vi "Position.vi"(0 "Position":dbl[][](array[numeric])) -> (6 "Position (output)":dbl[][](array[numeric]), 7 "Normalized Position":dbl[][](array[numeric]), 8 "RMS":dbl[][](array[numeric]), 9 "Pos, Neg increments Position":dbl[][](array[numeric]))   [LabVIEW 2020]
uses:
  <vilib>/Analysis/baseanly.llb/Mean (DBL).vi
  <vilib>/Analysis/5stat.llb/RMS (DBL).vi
  <vilib>/Analysis/NI_AALBase.lvlib
  <vilib>/Analysis/NI_AALPro.lvlib
panel:
  out "Positive, neg increments position":dbl[](array[numeric])
  out "Wrist Retraction":dbl
  out "Negative increments 6":dbl[](array[numeric])
  out "Wrist Protraction":dbl
  out "Positive increments 6":dbl[](array[numeric])
  out "Wrist Drop":dbl
  out "Negative increments 5":dbl[](array[numeric])
  out "Wrist Lift":dbl
  out "Positive increments 5":dbl[](array[numeric])
  out "Elbow Retraction":dbl
  out "Negative increments 4":dbl[](array[numeric])
  out "Elbow Protraction":dbl
  out "Positive increments 4":dbl[](array[numeric])
  out "Elbow Drop":dbl
  out "Negative increments 3":dbl[](array[numeric])
  out "Elbow Lift":dbl
  out "Positive increments 3":dbl[](array[numeric])
  out "Shoulder Retraction":dbl
  out "Negative increments 2":dbl[](array[numeric])
  out "Shoulder Protraction":dbl
  out "Positive increments 2":dbl[](array[numeric])
  out "Shoulder Drop":dbl
  out "Negative increments":dbl[](array[numeric])
  out "Shoulder Lift":dbl
  out "Positive increments":dbl[](array[numeric])
  out "size(s)":i32[](array[numeric])
  out "output array":dbl[](array[numeric])
  out "Array":dbl[][](array[numeric])
  out "Step Y (horizontal)":dbl[](graph)
  out "Step X (vertical)":dbl[](graph)
  out "Wrist X (vertical) 2":dbl[](graph)
  out "Wrist Y (horizontal) 2":dbl[](graph)
  out "Elbow X (vertical)  2":dbl[](graph)
  out "Elbow Y (horizontal)  2":dbl[](graph)
  out "Lower shoulder  X (vertical)  2":dbl[](graph)
  out "Lower shoulder Y (horizontal)  2":dbl[](graph)
  out "Upper shoulder X (vertical) 2":dbl[](graph)
  out "Upper shoulder Y (horizontal) 2":dbl[](graph)
  out "Wrist X (vertical)":dbl[](graph)
  out "Wrist Y (horizontal)":dbl[](graph)
  out "Elbow X (vertical)":dbl[](graph)
  out "Elbow Y (horizontal)":dbl[](graph)
  out "Lower shoulder  X (vertical)":dbl[](graph)
  out "Lower shoulder Y (horizontal)":dbl[](graph)
  out "Upper shoulder X (vertical)":dbl[](graph)
  out "Upper shoulder Y (horizontal)":dbl[](graph)
  # "Displacement and time kinematics"
  # "Upper Shoulder - Vertical"
  # "Upper shoulder - Horizontal"
  # "Lower Shoulder - Vertical"
  # "Lower shoulder - Horizontal"
  # "Elbow - Vertical"
  # "Elbow - Horizontal"
  # "Wrist - Vertical"
  # "Wrist - Horizontal"
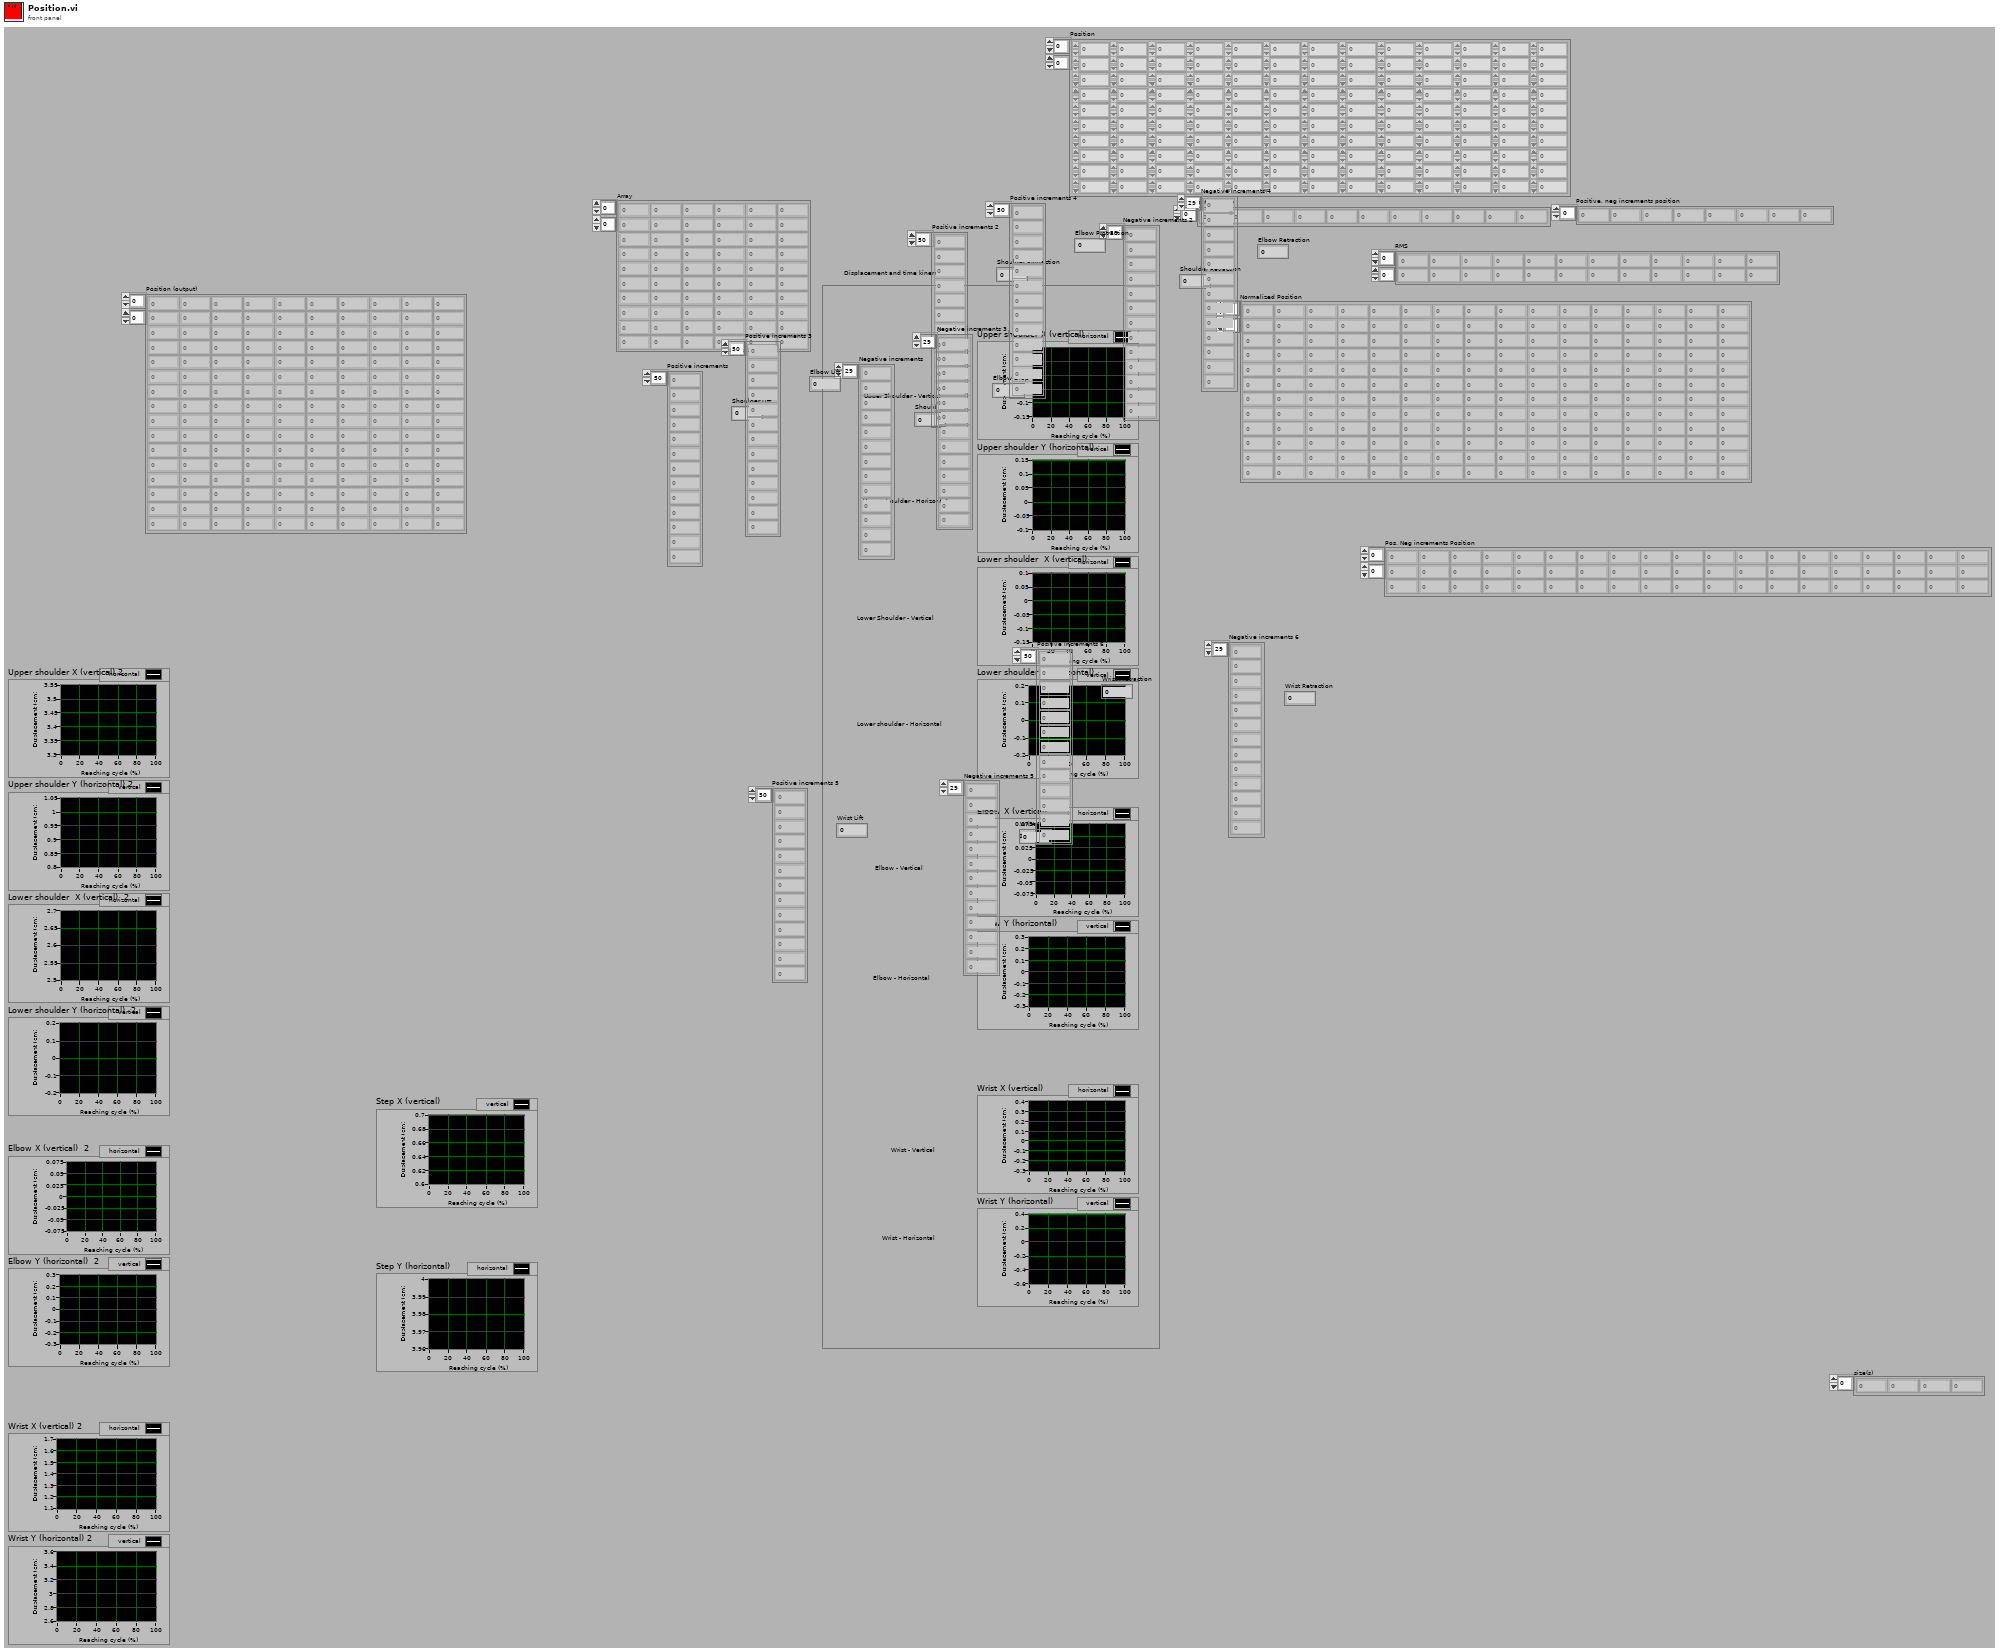
[diagram p1: front panel]
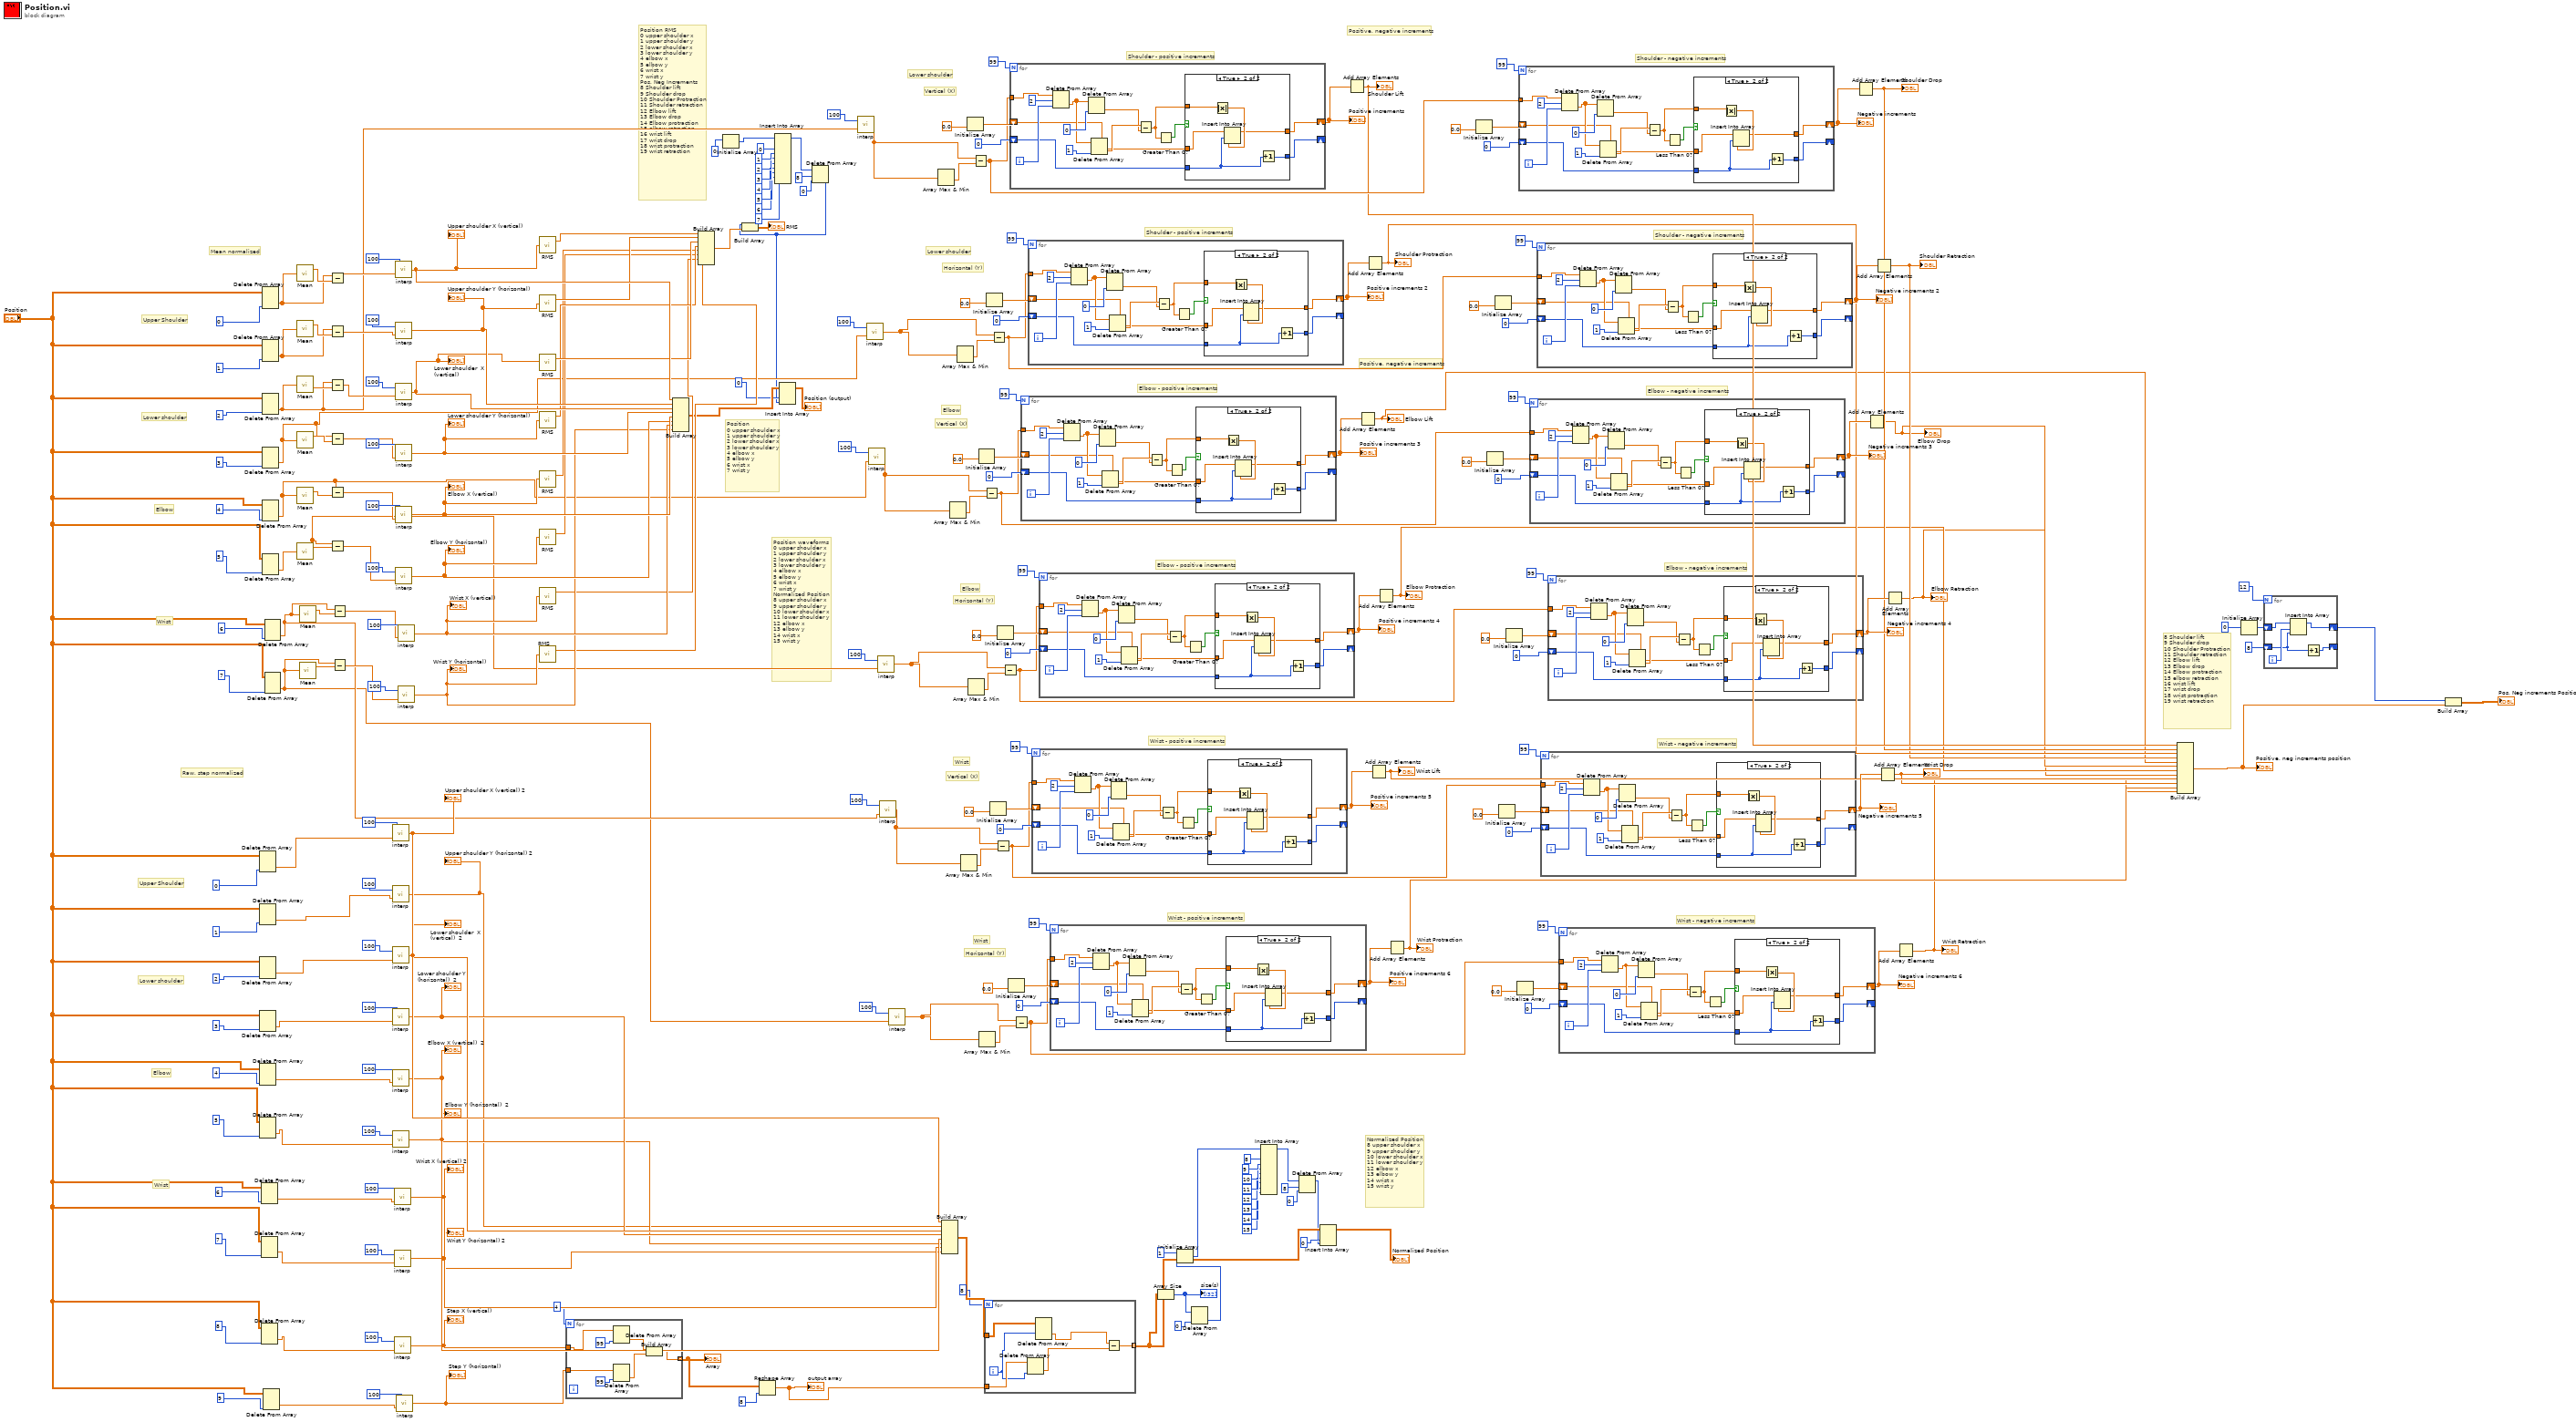
[diagram p0: block diagram]
diagram:
  # "Position waveforms\n0 upper shoulder x\n1 upper shoulder y\n2 lower shoulder x\n3 lower shoulder y\n4 elbow x\n5 elbow y\n6 wrist x\n7 wrist y\nNormalized Position\n8 upper shoulder x\n9 upper shoulder y\n10 lower shoulder x\n11 lower shoulder y\n12 elbow x\n13 elbow y\n14 wrist x\n15 wrist y"
  # "Position RMS\n0 upper shoulder x\n1 upper shoulder y\n2 lower shoulder x\n3 lower shoulder y\n4 elbow x\n5 elbow y\n6 wrist x\n7 wrist y\nPos, Neg Increments\n8 Shoulder lift\n9 Shoulder drop\n10 Shoulder Protraction\n11 Shoulder retraction\n12 Elbow lift\n13 Elbow drop\n14 Elbow protraction\n15 elbow retraction\n16 wrist lift\n17 wrist drop\n18 wrist protraction\n19 wrist retraction"
  # "8 Shoulder lift\n9 Shoulder drop\n10 Shoulder Protraction\n11 Shoulder retraction\n12 Elbow lift\n13 Elbow drop\n14 Elbow protraction\n15 elbow retraction\n16 wrist lift\n17 wrist drop\n18 wrist protraction\n19 wrist retraction"
  # "Wrist"
  # "Horizontal (Y)"
  # "Wrist - negative increments"
  # "Wrist - positive increments"
  # "Vertical (X)"
  # "Wrist - negative increments"
  # "Wrist - positive increments"
  # "Elbow"
  # "Horizontal (Y)"
  # "Elbow - negative increments"
  # "Elbow - positive increments"
  # "Vertical (X)"
  # "Elbow - negative increments"
  # "Elbow - positive increments"
  # "Positive, negative increments"
  # "Horizontal (Y)"
  # "Shoulder - negative increments"
  # "Shoulder - positive increments"
  # "Lower shoulder"
  # "Vertical (X)"
  # "Shoulder - negative increments"
  # "Shoulder - positive increments"
  # "Wrist"
  # "Elbow"
  # "Lower shoulder"
  # "Positive, negative increments"
  # "Normalized Position\n8 upper shoulder x\n9 upper shoulder y\n10 lower shoulder x\n11 lower shoulder y\n12 elbow x\n13 elbow y\n14 wrist x\n15 wrist y"
  # "Wrist"
  # "Elbow"
  # "Lower shoulder"
  # "Upper Shoulder"
  # "Raw, step normalized"
  # "Mean normalized"
  # "Wrist"
  # "Position\n0 upper shoulder x\n1 upper shoulder y\n2 lower shoulder x\n3 lower shoulder y\n4 elbow x\n5 elbow y\n6 wrist x\n7 wrist y"
  # "Elbow"
  # "Lower shoulder"
  # "Upper Shoulder"
  n1 = Delete From Array(array="Position", index (col)=0) -> (deleted portion=w189:dbl[])  [unwired: 2 in, 1 out]
  n2 = Delete From Array(array="Position", index (col)=1) -> (deleted portion=w188:dbl[])  [unwired: 2 in, 1 out]
  n3 = Delete From Array(array="Position", index (col)=2) -> (deleted portion=w187:dbl[])  [unwired: 2 in, 1 out]
  n4 = Delete From Array(array="Position", index (col)=3) -> (deleted portion=w186:dbl[])  [unwired: 2 in, 1 out]
  n5 = Delete From Array(array="Position", index (col)=4) -> (deleted portion=w185:dbl[])  [unwired: 2 in, 1 out]
  n6 = Delete From Array(array="Position", index (col)=5) -> (deleted portion=w184:dbl[])  [unwired: 2 in, 1 out]
  n7 = Delete From Array(array="Position", index (col)=6) -> (deleted portion=w183:dbl[])  [unwired: 2 in, 1 out]
  n8 = Delete From Array(array="Position", index (col)=7) -> (deleted portion=w182:dbl[])  [unwired: 2 in, 1 out]
  n9 = Delete From Array(array="Position", index (col)=8) -> (deleted portion=w176:dbl[])  [unwired: 2 in, 1 out]
  n10 = Delete From Array(array="Position", index (col)=0) -> (deleted portion=w131:dbl[])  [unwired: 2 in, 1 out]
  n11 = Delete From Array(array="Position", index (col)=1) -> (deleted portion=w222:dbl[])  [unwired: 2 in, 1 out]
  n12 = Delete From Array(array="Position", index (col)=2) -> (deleted portion=w114:dbl[])  [unwired: 2 in, 1 out]
  n13 = Delete From Array(array="Position", index (col)=3) -> (deleted portion=w99:dbl[])  [unwired: 2 in, 1 out]
  n14 = Delete From Array(array="Position", index (col)=4) -> (deleted portion=w69:dbl[])  [unwired: 2 in, 1 out]
  n15 = Delete From Array(array="Position", index (col)=5) -> (deleted portion=w68:dbl[])  [unwired: 2 in, 1 out]
  n16 = Delete From Array(array="Position", index (col)=9) -> (deleted portion=w175:dbl[])  [unwired: 2 in, 1 out]
  n17 = Delete From Array(array="Position", index (col)=6) -> (deleted portion=w39:dbl[])  [unwired: 2 in, 1 out]
  n18 = Delete From Array(array="Position", index (col)=7) -> (deleted portion=w38:dbl[])  [unwired: 2 in, 1 out]
  n19 = call-poly <vilib>:"Mean.vi"("X"=w131) -> ("mean"=w242:dbl)  [unwired: 1 out]
  n20 = call-poly <vilib>:"Mean.vi"("X"=w222) -> ("mean"=w243:dbl)  [unwired: 1 out]
  n21 = call-poly <vilib>:"Mean.vi"("X"=w114) -> ("mean"=w238:dbl)  [unwired: 1 out]
  n22 = call-poly <vilib>:"Mean.vi"("X"=w99) -> ("mean"=w239:dbl)  [unwired: 1 out]
  n23 = call-poly <vilib>:"Mean.vi"("X"=w69) -> ("mean"=w234:dbl)  [unwired: 1 out]
  n24 = call-poly <vilib>:"Mean.vi"("X"=w68) -> ("mean"=w235:dbl)  [unwired: 1 out]
  n25 = call-poly <vilib>:"Mean.vi"("X"=w39) -> ("mean"=w218:dbl)  [unwired: 1 out]
  n26 = call-poly <vilib>:"Mean.vi"("X"=w38) -> ("mean"=w219:dbl)  [unwired: 1 out]
  n27 = Subtract(x=w131, y=w242) -> (x-y=w130:dbl[])
  n28 = Subtract(x=w222, y=w243) -> (x-y=w227:dbl[])
  n29 = Subtract(x=w114, y=w238) -> (x-y=w226:dbl[])
  n30 = Subtract(x=w99, y=w239) -> (x-y=w225:dbl[])
  n31 = Subtract(x=w69, y=w234) -> (x-y=w224:dbl[])
  n32 = Subtract(x=w68, y=w235) -> (x-y=w223:dbl[])
  n33 = Subtract(x=w39, y=w218) -> (x-y=w215:dbl[])
  n34 = Subtract(x=w38, y=w219) -> (x-y=w214:dbl[])
  n35 = call "interp.vi"("first subarray"=w189, "nFRAMES"=100) -> ("emgInterp"=w201:dbl[])
  "Upper shoulder X (vertical) 2" <- w201
  n36 = call "interp.vi"("first subarray"=w188, "nFRAMES"=100) -> ("emgInterp"=w196:dbl[])
  "Upper shoulder Y (horizontal) 2" <- w196
  n37 = call "interp.vi"("first subarray"=w187, "nFRAMES"=100) -> ("emgInterp"=w200:dbl[])
  "Lower shoulder  X (vertical)  2" <- w200
  n38 = call "interp.vi"("first subarray"=w186, "nFRAMES"=100) -> ("emgInterp"=w199:dbl[])
  "Lower shoulder Y (horizontal)  2" <- w199
  n39 = call "interp.vi"("first subarray"=w185, "nFRAMES"=100) -> ("emgInterp"=w198:dbl[])
  "Elbow X (vertical)  2" <- w198
  n40 = call "interp.vi"("first subarray"=w184, "nFRAMES"=100) -> ("emgInterp"=w197:dbl[])
  "Elbow Y (horizontal)  2" <- w197
  n41 = call "interp.vi"("first subarray"=w183, "nFRAMES"=100) -> ("emgInterp"=w191:dbl[])
  "Wrist X (vertical) 2" <- w191
  n42 = call "interp.vi"("first subarray"=w182, "nFRAMES"=100) -> ("emgInterp"=w190:dbl[])
  "Wrist Y (horizontal) 2" <- w190
  n43 = call "interp.vi"("first subarray"=w176, "nFRAMES"=100) -> ("emgInterp"=w173:dbl[])
  "Step X (vertical)" <- w173
  n44 = call "interp.vi"("first subarray"=w130, "nFRAMES"=100) -> ("emgInterp"=w147:dbl[])
  "Upper shoulder X (vertical)" <- w147
  n45 = call "interp.vi"("first subarray"=w227, "nFRAMES"=100) -> ("emgInterp"=w146:dbl[])
  "Upper shoulder Y (horizontal)" <- w146
  n46 = call "interp.vi"("first subarray"=w226, "nFRAMES"=100) -> ("emgInterp"=w145:dbl[])
  "Lower shoulder  X (vertical)" <- w145
  n47 = call "interp.vi"("first subarray"=w225, "nFRAMES"=100) -> ("emgInterp"=w144:dbl[])
  "Lower shoulder Y (horizontal)" <- w144
  n48 = call "interp.vi"("first subarray"=w224, "nFRAMES"=100) -> ("emgInterp"=w143:dbl[])
  "Elbow X (vertical)" <- w143
  n49 = call "interp.vi"("first subarray"=w223, "nFRAMES"=100) -> ("emgInterp"=w142:dbl[])
  "Elbow Y (horizontal)" <- w142
  n50 = call "interp.vi"("first subarray"=w175, "nFRAMES"=100) -> ("emgInterp"=w172:dbl[])
  "Step Y (horizontal)" <- w172
  n51 = call "interp.vi"("first subarray"=w215, "nFRAMES"=100) -> ("emgInterp"=w141:dbl[])
  "Wrist X (vertical)" <- w141
  n52 = call "interp.vi"("first subarray"=w214, "nFRAMES"=100) -> ("emgInterp"=w140:dbl[])
  "Wrist Y (horizontal)" <- w140
  n53 = call-poly <vilib>:"RMS.vi"("X"=w147) -> ("rms value"=w139:dbl)  [unwired: 1 out]
  n54 = call-poly <vilib>:"RMS.vi"("X"=w146) -> ("rms value"=w138:dbl)  [unwired: 1 out]
  n55 = call-poly <vilib>:"RMS.vi"("X"=w145) -> ("rms value"=w137:dbl)  [unwired: 1 out]
  n56 = call-poly <vilib>:"RMS.vi"("X"=w144) -> ("rms value"=w136:dbl)  [unwired: 1 out]
  n57 = call-poly <vilib>:"RMS.vi"("X"=w143) -> ("rms value"=w135:dbl)  [unwired: 1 out]
  n58 = call-poly <vilib>:"RMS.vi"("X"=w142) -> ("rms value"=w134:dbl)  [unwired: 1 out]
  n59 = call-poly <vilib>:"RMS.vi"("X"=w141) -> ("rms value"=w133:dbl)  [unwired: 1 out]
  n60 = call-poly <vilib>:"RMS.vi"("X"=w140) -> ("rms value"=w132:dbl)  [unwired: 1 out]
  n61 = for {
    N: 4 -> [_]
    tunnel: w173 -> [w247]
    tunnel: [w248] -> w170 mode=indexing
    tunnel: w172 -> [w246]
    n62 = Delete From Array(array=w247, index=99) -> (deleted portion=w250:dbl)  [unwired: 1 in, 1 out]
    n63 = Delete From Array(array=w246, index=99) -> (deleted portion=w249:dbl)  [unwired: 1 in, 1 out]
    n64 = Build Array(w250, w249) -> (w248:dbl[])
  }
  "Array" <- w170
  n65 = Build Array(w147, w146, w145, w144, w143, w142, w141, w140) -> (w18:dbl[][])
  n66 = Build Array(w139, w138, w137, w136, w135, w134, w133, w132) -> (w129:dbl[])
  n67 = Initialize Array(0) -> (w3:i32[])  [unwired: 1 in]
  n68 = Reshape Array(w170, 8) -> (w168:dbl[])
  "output array" <- w168
  n69 = Insert Into Array(array=w3, new element #1=0, new element #2=1, new element #3=2, new element #4=3, new element #5=4, new element #6=5, new element #7=6, new element #8=7) -> (w7:i32[])  [unwired: 1 in]
  n70 = Delete From Array(array=w7, length=8, index=0) -> (deleted portion=w1:i32[])  [unwired: 1 out]
  n71 = Build Array(w1, w129) -> (→"RMS":dbl[][])
  n72 = Insert Into Array(array=w18, index (col)=0, new element=w1) -> (→"Position (output)":dbl[][])  [unwired: 1 in]
  n73 = call "interp.vi"("first subarray"=w114, "nFRAMES"=100) -> ("emgInterp"=w113:dbl[])
  n74 = call "interp.vi"("first subarray"=w99, "nFRAMES"=100) -> ("emgInterp"=w98:dbl[])
  n75 = call "interp.vi"("first subarray"=w69, "nFRAMES"=100) -> ("emgInterp"=w84:dbl[])
  n76 = call "interp.vi"("first subarray"=w68, "nFRAMES"=100) -> ("emgInterp"=w70:dbl[])
  n77 = call "interp.vi"("first subarray"=w39, "nFRAMES"=100) -> ("emgInterp"=w54:dbl[])
  n78 = call "interp.vi"("first subarray"=w38, "nFRAMES"=100) -> ("emgInterp"=w40:dbl[])
  n79 = Array Max & Min(array=w113) -> (min value=w127:dbl)  [unwired: 3 out]
  n80 = Build Array(w201, w196, w200, w199, w198, w197, w191, w190) -> (w169:dbl[][])
  n81 = Array Max & Min(array=w84) -> (min value=w97:dbl)  [unwired: 3 out]
  n82 = Array Max & Min(array=w98) -> (min value=w112:dbl)  [unwired: 3 out]
  n83 = Array Max & Min(array=w54) -> (min value=w67:dbl)  [unwired: 3 out]
  n84 = Initialize Array(0.0) -> (w125:dbl[])  [unwired: 1 in]
  n85 = Array Max & Min(array=w70) -> (min value=w83:dbl)  [unwired: 3 out]
  n86 = Subtract(x=w113, y=w127) -> (x-y=w116:dbl[])
  n87 = Initialize Array(0.0) -> (w95:dbl[])  [unwired: 1 in]
  n88 = Array Max & Min(array=w40) -> (min value=w53:dbl)  [unwired: 3 out]
  n89 = Subtract(x=w84, y=w97) -> (x-y=w86:dbl[])
  n90 = for {
    N: 8 -> [_]
    tunnel: w169 -> [w258]
    tunnel: [w256] -> w149 mode=indexing
    tunnel: w168 -> [w255]
    i -> [w254]
    n91 = Delete From Array(array=w255, index=w254) -> (deleted portion=w253:dbl)  [unwired: 1 in, 1 out]
    n92 = Delete From Array(array=w258, index (row)=w254) -> (deleted portion=w257:dbl[])  [unwired: 2 in, 1 out]
    n93 = Subtract(x=w257, y=w253) -> (x-y=w256:dbl[])
  }
  n94 = Initialize Array(0.0) -> (w110:dbl[])  [unwired: 1 in]
  n95 = Initialize Array(0.0) -> (w65:dbl[])  [unwired: 1 in]
  n96 = Subtract(x=w98, y=w112) -> (x-y=w101:dbl[])
  n97 = Subtract(x=w54, y=w67) -> (x-y=w56:dbl[])
  n98 = Initialize Array(0.0) -> (w81:dbl[])  [unwired: 1 in]
  n99 = Subtract(x=w70, y=w83) -> (x-y=w72:dbl[])
  n100 = Initialize Array(0.0) -> (w51:dbl[])  [unwired: 1 in]
  n101 = for {
    N: 99 -> [_]
    shift-right: [w259] -> _
    shift-left: 0 -> [w261]
    shift-right: [w260] -> w122
    shift-left: w125 -> [w262]
    tunnel: w116 -> [w272]
    i -> [w271]
    n102 = Delete From Array(array=w272, length=2, index=w271) -> (deleted portion=w267:dbl[])  [unwired: 1 out]
    n103 = Delete From Array(array=w267, index=0) -> (deleted portion=w265:dbl)  [unwired: 1 in, 1 out]
    n104 = Delete From Array(array=w267, index=1) -> (deleted portion=w266:dbl)  [unwired: 1 in, 1 out]
    n105 = Subtract(x=w266, y=w265) -> (x-y=w263:dbl)
    n106 = Greater Than 0?(x=w263) -> (x > 0?=w264:bool)
    n107 = case shown="True" w264 {
      tunnel: w263 -> [_ w280]
      tunnel: w262 -> [w274 w279]
      tunnel: w261 -> [w273 w276]
      tunnel: [w274 w277] -> w260
      tunnel: [w273 w275] -> w259
      frame False {
      }
      frame True {
        n108 = Absolute Value(x=w280) -> (abs(x)=w278:dbl)
        n109 = Insert Into Array(array=w279, index=w276, new element=w278) -> (w277:dbl[])
        n110 = Increment(x=w276) -> (x+1=w275:i32)
      }
    }
  }
  "Positive increments" <- w122
  n111 = Subtract(x=w40, y=w53) -> (x-y=w42:dbl[])
  n112 = for {
    N: 99 -> [_]
    shift-right: [w281] -> _
    shift-left: 0 -> [w283]
    shift-right: [w282] -> w92
    shift-left: w95 -> [w284]
    tunnel: w86 -> [w294]
    i -> [w293]
    n113 = Delete From Array(array=w294, length=2, index=w293) -> (deleted portion=w289:dbl[])  [unwired: 1 out]
    n114 = Delete From Array(array=w289, index=0) -> (deleted portion=w287:dbl)  [unwired: 1 in, 1 out]
    n115 = Delete From Array(array=w289, index=1) -> (deleted portion=w288:dbl)  [unwired: 1 in, 1 out]
    n116 = Subtract(x=w288, y=w287) -> (x-y=w285:dbl)
    n117 = Greater Than 0?(x=w285) -> (x > 0?=w286:bool)
    n118 = case shown="True" w286 {
      tunnel: w285 -> [_ w302]
      tunnel: w284 -> [w296 w301]
      tunnel: w283 -> [w295 w298]
      tunnel: [w296 w299] -> w282
      tunnel: [w295 w297] -> w281
      frame False {
      }
      frame True {
        n119 = Absolute Value(x=w302) -> (abs(x)=w300:dbl)
        n120 = Insert Into Array(array=w301, index=w298, new element=w300) -> (w299:dbl[])
        n121 = Increment(x=w298) -> (x+1=w297:i32)
      }
    }
  }
  "Positive increments 3" <- w92
  n122 = for {
    N: 99 -> [_]
    shift-right: [w303] -> _
    shift-left: 0 -> [w305]
    shift-right: [w304] -> w107
    shift-left: w110 -> [w306]
    tunnel: w101 -> [w316]
    i -> [w315]
    n123 = Delete From Array(array=w316, length=2, index=w315) -> (deleted portion=w311:dbl[])  [unwired: 1 out]
    n124 = Delete From Array(array=w311, index=0) -> (deleted portion=w309:dbl)  [unwired: 1 in, 1 out]
    n125 = Delete From Array(array=w311, index=1) -> (deleted portion=w310:dbl)  [unwired: 1 in, 1 out]
    n126 = Subtract(x=w310, y=w309) -> (x-y=w307:dbl)
    n127 = Greater Than 0?(x=w307) -> (x > 0?=w308:bool)
    n128 = case shown="True" w308 {
      tunnel: w307 -> [_ w324]
      tunnel: w306 -> [w318 w323]
      tunnel: w305 -> [w317 w320]
      tunnel: [w318 w321] -> w304
      tunnel: [w317 w319] -> w303
      frame False {
      }
      frame True {
        n129 = Absolute Value(x=w324) -> (abs(x)=w322:dbl)
        n130 = Insert Into Array(array=w323, index=w320, new element=w322) -> (w321:dbl[])
        n131 = Increment(x=w320) -> (x+1=w319:i32)
      }
    }
  }
  "Positive increments 2" <- w107
  n132 = for {
    N: 99 -> [_]
    shift-right: [w325] -> _
    shift-left: 0 -> [w327]
    shift-right: [w326] -> w62
    shift-left: w65 -> [w328]
    tunnel: w56 -> [w338]
    i -> [w337]
    n133 = Delete From Array(array=w338, length=2, index=w337) -> (deleted portion=w333:dbl[])  [unwired: 1 out]
    n134 = Delete From Array(array=w333, index=0) -> (deleted portion=w331:dbl)  [unwired: 1 in, 1 out]
    n135 = Delete From Array(array=w333, index=1) -> (deleted portion=w332:dbl)  [unwired: 1 in, 1 out]
    n136 = Subtract(x=w332, y=w331) -> (x-y=w329:dbl)
    n137 = Greater Than 0?(x=w329) -> (x > 0?=w330:bool)
    n138 = case shown="True" w330 {
      tunnel: w329 -> [_ w346]
      tunnel: w328 -> [w340 w345]
      tunnel: w327 -> [w339 w342]
      tunnel: [w340 w343] -> w326
      tunnel: [w339 w341] -> w325
      frame False {
      }
      frame True {
        n139 = Absolute Value(x=w346) -> (abs(x)=w344:dbl)
        n140 = Insert Into Array(array=w345, index=w342, new element=w344) -> (w343:dbl[])
        n141 = Increment(x=w342) -> (x+1=w341:i32)
      }
    }
  }
  "Positive increments 5" <- w62
  n142 = for {
    N: 99 -> [_]
    shift-right: [w347] -> _
    shift-left: 0 -> [w349]
    shift-right: [w348] -> w78
    shift-left: w81 -> [w350]
    tunnel: w72 -> [w360]
    i -> [w359]
    n143 = Delete From Array(array=w360, length=2, index=w359) -> (deleted portion=w355:dbl[])  [unwired: 1 out]
    n144 = Delete From Array(array=w355, index=0) -> (deleted portion=w353:dbl)  [unwired: 1 in, 1 out]
    n145 = Delete From Array(array=w355, index=1) -> (deleted portion=w354:dbl)  [unwired: 1 in, 1 out]
    n146 = Subtract(x=w354, y=w353) -> (x-y=w351:dbl)
    n147 = Greater Than 0?(x=w351) -> (x > 0?=w352:bool)
    n148 = case shown="True" w352 {
      tunnel: w351 -> [_ w368]
      tunnel: w350 -> [w362 w367]
      tunnel: w349 -> [w361 w364]
      tunnel: [w362 w365] -> w348
      tunnel: [w361 w363] -> w347
      frame False {
      }
      frame True {
        n149 = Absolute Value(x=w368) -> (abs(x)=w366:dbl)
        n150 = Insert Into Array(array=w367, index=w364, new element=w366) -> (w365:dbl[])
        n151 = Increment(x=w364) -> (x+1=w363:i32)
      }
    }
  }
  "Positive increments 4" <- w78
  n152 = for {
    N: 99 -> [_]
    shift-right: [w369] -> _
    shift-left: 0 -> [w371]
    shift-right: [w370] -> w48
    shift-left: w51 -> [w372]
    tunnel: w42 -> [w382]
    i -> [w381]
    n153 = Delete From Array(array=w382, length=2, index=w381) -> (deleted portion=w377:dbl[])  [unwired: 1 out]
    n154 = Delete From Array(array=w377, index=0) -> (deleted portion=w375:dbl)  [unwired: 1 in, 1 out]
    n155 = Delete From Array(array=w377, index=1) -> (deleted portion=w376:dbl)  [unwired: 1 in, 1 out]
    n156 = Subtract(x=w376, y=w375) -> (x-y=w373:dbl)
    n157 = Greater Than 0?(x=w373) -> (x > 0?=w374:bool)
    n158 = case shown="True" w374 {
      tunnel: w373 -> [_ w390]
      tunnel: w372 -> [w384 w389]
      tunnel: w371 -> [w383 w386]
      tunnel: [w384 w387] -> w370
      tunnel: [w383 w385] -> w369
      frame False {
      }
      frame True {
        n159 = Absolute Value(x=w390) -> (abs(x)=w388:dbl)
        n160 = Insert Into Array(array=w389, index=w386, new element=w388) -> (w387:dbl[])
        n161 = Increment(x=w386) -> (x+1=w385:i32)
      }
    }
  }
  "Positive increments 6" <- w48
  n162 = Array Size(array=w149) -> (size(s)=w153:i32[])
  "size(s)" <- w153
  n163 = Delete From Array(array=w153, index=0) -> (deleted portion=w151:i32)  [unwired: 1 in, 1 out]
  n164 = Initialize Array(1, w151) -> (w165:i32[])
  n165 = Insert Into Array(array=w165, new element #1=8, new element #2=9, new element #3=10, new element #4=11, new element #5=12, new element #6=13, new element #7=14, new element #8=15) -> (w156:i32[])  [unwired: 1 in]
  n166 = Delete From Array(array=w156, length=8, index=0) -> (array with subset deleted=w17:i32[])  [unwired: 1 out]
  n167 = Insert Into Array(array=w149, index (col)=0, new element=w17) -> (→"Normalized Position":dbl[][])  [unwired: 1 in]
  n168 = Add Array Elements(numeric array=w122) -> (sum=w37:dbl)
  "Shoulder Lift" <- w37
  n169 = Add Array Elements(numeric array=w92) -> (sum=w33:dbl)
  "Elbow Lift" <- w33
  n170 = Add Array Elements(numeric array=w107) -> (sum=w35:dbl)
  "Shoulder Protraction" <- w35
  n171 = Add Array Elements(numeric array=w62) -> (sum=w29:dbl)
  "Wrist Lift" <- w29
  n172 = Add Array Elements(numeric array=w78) -> (sum=w31:dbl)
  "Elbow Protraction" <- w31
  n173 = Add Array Elements(numeric array=w48) -> (sum=w27:dbl)
  "Wrist Protraction" <- w27
  n174 = Initialize Array(0.0) -> (w120:dbl[])  [unwired: 1 in]
  n175 = Initialize Array(0.0) -> (w90:dbl[])  [unwired: 1 in]
  n176 = Initialize Array(0.0) -> (w105:dbl[])  [unwired: 1 in]
  n177 = Initialize Array(0.0) -> (w60:dbl[])  [unwired: 1 in]
  n178 = Initialize Array(0.0) -> (w76:dbl[])  [unwired: 1 in]
  n179 = Initialize Array(0.0) -> (w46:dbl[])  [unwired: 1 in]
  n180 = for {
    N: 99 -> [_]
    shift-right: [w391] -> _
    shift-left: 0 -> [w393]
    shift-right: [w392] -> w117
    shift-left: w120 -> [w394]
    tunnel: w116 -> [w404]
    i -> [w403]
    n181 = Delete From Array(array=w404, length=2, index=w403) -> (deleted portion=w399:dbl[])  [unwired: 1 out]
    n182 = Delete From Array(array=w399, index=0) -> (deleted portion=w397:dbl)  [unwired: 1 in, 1 out]
    n183 = Delete From Array(array=w399, index=1) -> (deleted portion=w398:dbl)  [unwired: 1 in, 1 out]
    n184 = Subtract(x=w398, y=w397) -> (x-y=w395:dbl)
    n185 = Less Than 0?(x=w395) -> (x < 0?=w396:bool)
    n186 = case shown="True" w396 {
      tunnel: w395 -> [_ w412]
      tunnel: w394 -> [w406 w411]
      tunnel: w393 -> [w405 w408]
      tunnel: [w406 w409] -> w392
      tunnel: [w405 w407] -> w391
      frame False {
      }
      frame True {
        n187 = Absolute Value(x=w412) -> (abs(x)=w410:dbl)
        n188 = Insert Into Array(array=w411, index=w408, new element=w410) -> (w409:dbl[])
        n189 = Increment(x=w408) -> (x+1=w407:i32)
      }
    }
  }
  "Negative increments" <- w117
  n190 = for {
    N: 99 -> [_]
    shift-right: [w413] -> _
    shift-left: 0 -> [w415]
    shift-right: [w414] -> w87
    shift-left: w90 -> [w416]
    tunnel: w86 -> [w426]
    i -> [w425]
    n191 = Delete From Array(array=w426, length=2, index=w425) -> (deleted portion=w421:dbl[])  [unwired: 1 out]
    n192 = Delete From Array(array=w421, index=0) -> (deleted portion=w419:dbl)  [unwired: 1 in, 1 out]
    n193 = Delete From Array(array=w421, index=1) -> (deleted portion=w420:dbl)  [unwired: 1 in, 1 out]
    n194 = Subtract(x=w420, y=w419) -> (x-y=w417:dbl)
    n195 = Less Than 0?(x=w417) -> (x < 0?=w418:bool)
    n196 = case shown="True" w418 {
      tunnel: w417 -> [_ w434]
      tunnel: w416 -> [w428 w433]
      tunnel: w415 -> [w427 w430]
      tunnel: [w428 w431] -> w414
      tunnel: [w427 w429] -> w413
      frame False {
      }
      frame True {
        n197 = Absolute Value(x=w434) -> (abs(x)=w432:dbl)
        n198 = Insert Into Array(array=w433, index=w430, new element=w432) -> (w431:dbl[])
        n199 = Increment(x=w430) -> (x+1=w429:i32)
      }
    }
  }
  "Negative increments 3" <- w87
  n200 = for {
    N: 99 -> [_]
    shift-right: [w435] -> _
    shift-left: 0 -> [w437]
    shift-right: [w436] -> w102
    shift-left: w105 -> [w438]
    tunnel: w101 -> [w448]
    i -> [w447]
    n201 = Delete From Array(array=w448, length=2, index=w447) -> (deleted portion=w443:dbl[])  [unwired: 1 out]
    n202 = Delete From Array(array=w443, index=0) -> (deleted portion=w441:dbl)  [unwired: 1 in, 1 out]
    n203 = Delete From Array(array=w443, index=1) -> (deleted portion=w442:dbl)  [unwired: 1 in, 1 out]
    n204 = Subtract(x=w442, y=w441) -> (x-y=w439:dbl)
    n205 = Less Than 0?(x=w439) -> (x < 0?=w440:bool)
    n206 = case shown="True" w440 {
      tunnel: w439 -> [_ w456]
      tunnel: w438 -> [w450 w455]
      tunnel: w437 -> [w449 w452]
      tunnel: [w450 w453] -> w436
      tunnel: [w449 w451] -> w435
      frame False {
      }
      frame True {
        n207 = Absolute Value(x=w456) -> (abs(x)=w454:dbl)
        n208 = Insert Into Array(array=w455, index=w452, new element=w454) -> (w453:dbl[])
        n209 = Increment(x=w452) -> (x+1=w451:i32)
      }
    }
  }
  "Negative increments 2" <- w102
  n210 = for {
    N: 99 -> [_]
    shift-right: [w457] -> _
    shift-left: 0 -> [w459]
    shift-right: [w458] -> w57
    shift-left: w60 -> [w460]
    tunnel: w56 -> [w470]
    i -> [w469]
    n211 = Delete From Array(array=w470, length=2, index=w469) -> (deleted portion=w465:dbl[])  [unwired: 1 out]
    n212 = Delete From Array(array=w465, index=0) -> (deleted portion=w463:dbl)  [unwired: 1 in, 1 out]
    n213 = Delete From Array(array=w465, index=1) -> (deleted portion=w464:dbl)  [unwired: 1 in, 1 out]
    n214 = Subtract(x=w464, y=w463) -> (x-y=w461:dbl)
    n215 = Less Than 0?(x=w461) -> (x < 0?=w462:bool)
    n216 = case shown="True" w462 {
      tunnel: w461 -> [_ w478]
      tunnel: w460 -> [w472 w477]
      tunnel: w459 -> [w471 w474]
      tunnel: [w472 w475] -> w458
      tunnel: [w471 w473] -> w457
      frame False {
      }
      frame True {
        n217 = Absolute Value(x=w478) -> (abs(x)=w476:dbl)
        n218 = Insert Into Array(array=w477, index=w474, new element=w476) -> (w475:dbl[])
        n219 = Increment(x=w474) -> (x+1=w473:i32)
      }
    }
  }
  "Negative increments 5" <- w57
  n220 = for {
    N: 99 -> [_]
    shift-right: [w479] -> _
    shift-left: 0 -> [w481]
    shift-right: [w480] -> w73
    shift-left: w76 -> [w482]
    tunnel: w72 -> [w492]
    i -> [w491]
    n221 = Delete From Array(array=w492, length=2, index=w491) -> (deleted portion=w487:dbl[])  [unwired: 1 out]
    n222 = Delete From Array(array=w487, index=0) -> (deleted portion=w485:dbl)  [unwired: 1 in, 1 out]
    n223 = Delete From Array(array=w487, index=1) -> (deleted portion=w486:dbl)  [unwired: 1 in, 1 out]
    n224 = Subtract(x=w486, y=w485) -> (x-y=w483:dbl)
    n225 = Less Than 0?(x=w483) -> (x < 0?=w484:bool)
    n226 = case shown="True" w484 {
      tunnel: w483 -> [_ w500]
      tunnel: w482 -> [w494 w499]
      tunnel: w481 -> [w493 w496]
      tunnel: [w494 w497] -> w480
      tunnel: [w493 w495] -> w479
      frame False {
      }
      frame True {
        n227 = Absolute Value(x=w500) -> (abs(x)=w498:dbl)
        n228 = Insert Into Array(array=w499, index=w496, new element=w498) -> (w497:dbl[])
        n229 = Increment(x=w496) -> (x+1=w495:i32)
      }
    }
  }
  "Negative increments 4" <- w73
  n230 = for {
    N: 99 -> [_]
    shift-right: [w501] -> _
    shift-left: 0 -> [w503]
    shift-right: [w502] -> w43
    shift-left: w46 -> [w504]
    tunnel: w42 -> [w514]
    i -> [w513]
    n231 = Delete From Array(array=w514, length=2, index=w513) -> (deleted portion=w509:dbl[])  [unwired: 1 out]
    n232 = Delete From Array(array=w509, index=0) -> (deleted portion=w507:dbl)  [unwired: 1 in, 1 out]
    n233 = Delete From Array(array=w509, index=1) -> (deleted portion=w508:dbl)  [unwired: 1 in, 1 out]
    n234 = Subtract(x=w508, y=w507) -> (x-y=w505:dbl)
    n235 = Less Than 0?(x=w505) -> (x < 0?=w506:bool)
    n236 = case shown="True" w506 {
      tunnel: w505 -> [_ w522]
      tunnel: w504 -> [w516 w521]
      tunnel: w503 -> [w515 w518]
      tunnel: [w516 w519] -> w502
      tunnel: [w515 w517] -> w501
      frame False {
      }
      frame True {
        n237 = Absolute Value(x=w522) -> (abs(x)=w520:dbl)
        n238 = Insert Into Array(array=w521, index=w518, new element=w520) -> (w519:dbl[])
        n239 = Increment(x=w518) -> (x+1=w517:i32)
      }
    }
  }
  "Negative increments 6" <- w43
  n240 = Add Array Elements(numeric array=w117) -> (sum=w36:dbl)
  "Shoulder Drop" <- w36
  n241 = Add Array Elements(numeric array=w87) -> (sum=w32:dbl)
  "Elbow Drop" <- w32
  n242 = Add Array Elements(numeric array=w102) -> (sum=w34:dbl)
  "Shoulder Retraction" <- w34
  n243 = Add Array Elements(numeric array=w57) -> (sum=w28:dbl)
  "Wrist Drop" <- w28
  n244 = Add Array Elements(numeric array=w73) -> (sum=w30:dbl)
  "Elbow Retraction" <- w30
  n245 = Add Array Elements(numeric array=w43) -> (sum=w26:dbl)
  "Wrist Retraction" <- w26
  n246 = Build Array(w37, w36, w35, w34, w33, w32, w31, w30, w29, w28, w27, w26) -> (w20:dbl[])
  "Positive, neg increments position" <- w20
  n247 = Initialize Array(0) -> (w23:i32[])  [unwired: 1 in]
  n248 = for {
    N: 12 -> [_]
    shift-right: [w525] -> w21
    shift-left: w23 -> [w526]
    shift-right: [w523] -> _
    shift-left: 8 -> [w524]
    i -> [w527]
    n249 = Insert Into Array(array=w526, index=w527, new element=w524) -> (w525:i32[])
    n250 = Increment(x=w524) -> (x+1=w523:i32)
  }
  n251 = Build Array(w21, w20) -> (→"Pos, Neg increments Position":dbl[][])
